vi "NEVSTOP QD Shortcuts.vi"(6 "Variant in":variant, 7 "Shift Pressed?":bool, 8 "error in (no error)":errorcluster, 10 "QD Combo Box Ref":refnum<vi>, 11 "QD Launch VI Ref":refnum<vi>) -> (0 "error out":errorcluster, 4 "Variant out":variant)   [LabVIEW 2017, in "NEVSTOP QD Shortcuts.lvlib"]
doc: "NEVSTOP Quickdrops. Using a choosing dialog for quick QD selection.\n\nDefault Shortcut - [Q]"
uses:
  NEVSTOP QD Shortcuts.lvlib
panel:
  in  "Undo Name":string="NESTOP Shortcuts"
  # "Do not change the connector pane of this VI.\n\nSee the block diagram for directions on how to use this template."
  # "Specify the name of the Undo transaction"
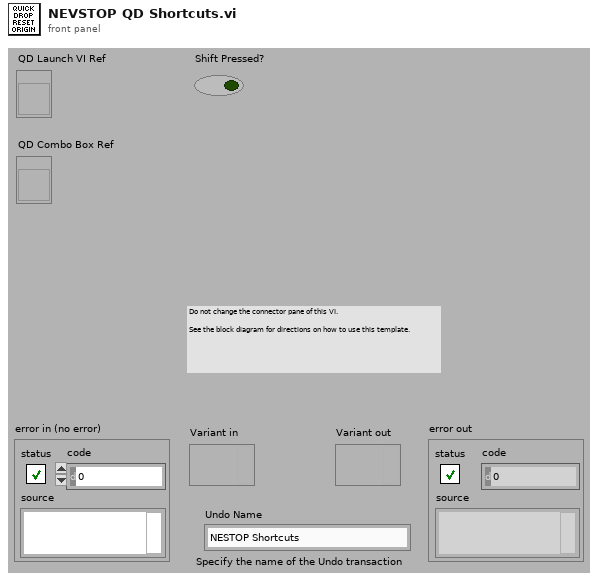
[diagram p1: front panel]
types:
  T1 = typedef "QuickDrop QDKS Info.ctl" = cluster{"VI Name":string, "VI Path":path, "Default Shortcut":string, "Assigned Shortcut":string, "Description":string}
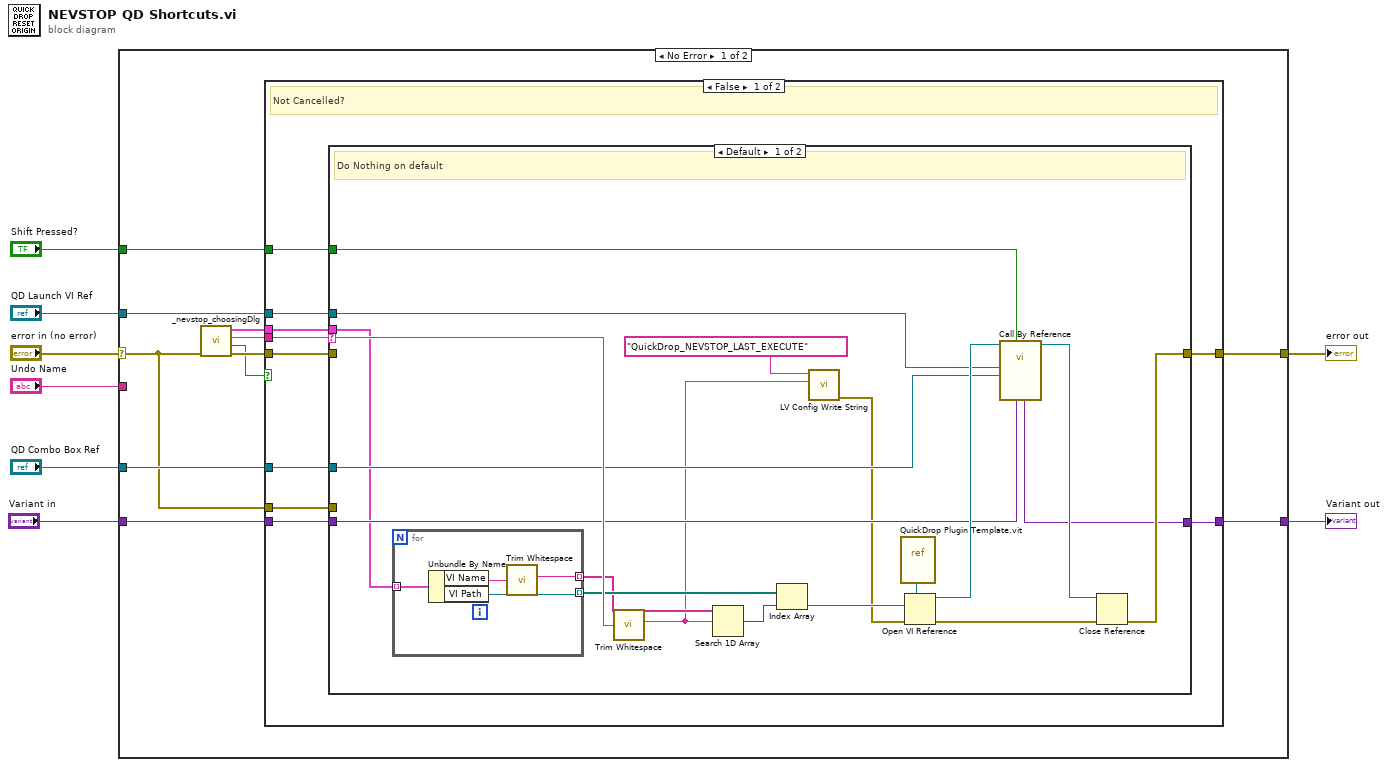
[diagram p0: block diagram]
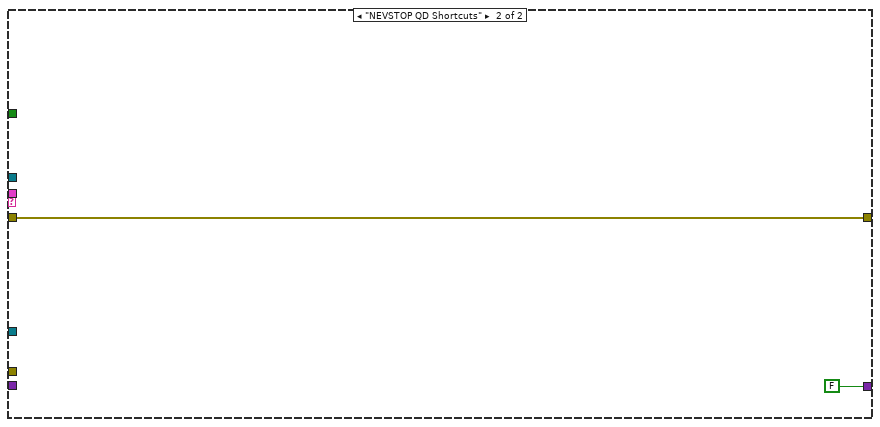
[diagram p2: hidden frame]
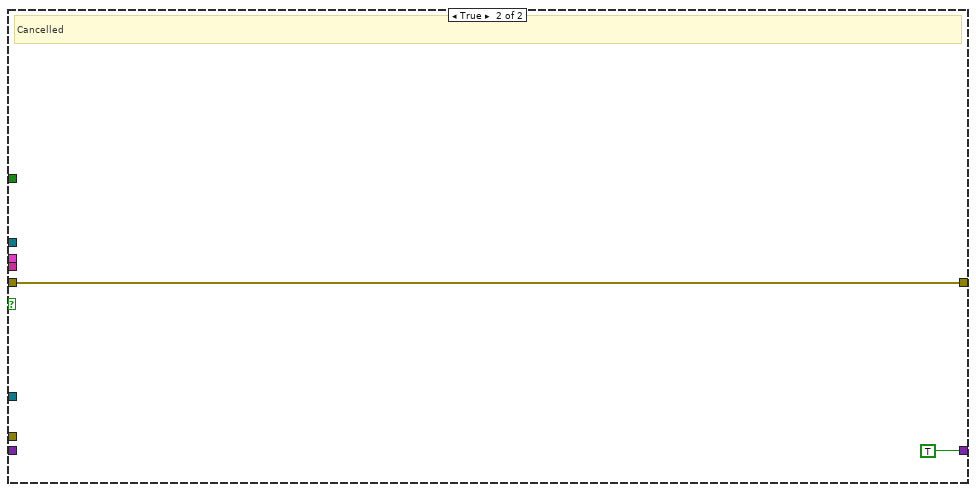
[diagram p3: hidden frame]
diagram:
  n1 = case shown="No Error" "error in (no error)" {
    selector: "error in (no error)" -> [w10 w57]
    tunnel: [w14 w57] -> w7
    tunnel: "QD Launch VI Ref" -> [w13 _]
    tunnel: "Shift Pressed?" -> [w17 _]
    tunnel: "QD Combo Box Ref" -> [w16 _]
    tunnel: "Variant in" -> [w12 _]
    tunnel: "Undo Name" -> [_ _]
    tunnel: [w11 _] -> w1
    frame No Error {
      n2 = call "_nevstop_choosingDlg.vi"("error in (no error)"=w10) -> ("error out"=w18:errorcluster, "Cancelled?"=w15:bool, "QuckDrop"=w19:string, "QDKS Info"=w9:T1[])  [unwired: 6 in, 1 out]
      n3 = case shown="False" w15 {
        tunnel: w19 -> [w29 _]
        tunnel: w18 -> [w28 w56]
        tunnel: w17 -> [w27 _]
        tunnel: w16 -> [w26 _]
        tunnel: [w25 w56] -> w14
        tunnel: w13 -> [w24 _]
        tunnel: w12 -> [w23 _]
        tunnel: [w22 TRUE] -> w11
        tunnel: w10 -> [w21 _]
        tunnel: w9 -> [w20 _]
        frame False {
          # "Not Cancelled?"
          n4 = case shown="Default" w29 {
            selector: w29 -> [w47 _]
            tunnel: w28 -> [_ w54]
            tunnel: w27 -> [w37 _]
            tunnel: w26 -> [w38 _]
            tunnel: [w41 w54] -> w25
            tunnel: w24 -> [w39 _]
            tunnel: w23 -> [w40 _]
            tunnel: [w36 FALSE] -> w22
            tunnel: w21 -> [_ _]
            tunnel: w20 -> [w33 _]
            frame Default {
              # "Do Nothing on default"
              n5 = for {
                tunnel: w33 -> [w52] mode=indexing
                tunnel: [w49] -> w34 mode=indexing
                tunnel: [w50] -> w46 mode=indexing
                n6 = Unbundle By Name(w52) -> ("VI Name"=w51:string, "VI Path"=w50:path)
                n7 = call-poly <vilib>:"Trim Whitespace.vi"("string"=w51) -> ("trimmed string"=w49:string)  [unwired: 1 in]
              }
              n8 = call-poly <vilib>:"Trim Whitespace.vi"("string"=w47) -> ("trimmed string"=w31:string)  [unwired: 1 in]
              n9 = Search 1D Array(1D array=w34, element=w31) -> (index of element=w45:i32)  [unwired: 1 in]
              n10 = Index Array(array=w46, index=w45) -> (element=w44:path)
              n11 = call <resource>:"LV Config Write String.vi"("value"=w31, "key"="QuickDrop_NEVSTOP_LAST_EXECUTE") -> ("error out"=w30:errorcluster)  [unwired: 5 in]
              n12 = vi-ref <resource>:"QuickDrop Plugin Template.vit"() -> (w48:refnum<vi>)
              n13 = Open VI Reference(type specifier VI Refnum (for type only)=w48, vi path=w44, error in (no error)=w30) -> (vi reference=w43:refnum<vi>, error out=w35:errorcluster)  [unwired: 3 in]
              n14 = call-by-ref "?"(reference=w43, "Variant in"=w40, "Shift Pressed?"=w37, "QD Combo Box Ref"=w38, "QD Launch VI Ref"=w39) -> (reference out=w42:refnum<vi>, "Variant out"=w36:variant)  [unwired: 7 in, 2 out]
              n15 = Close Reference(reference=w42, error in (no error)=w35) -> (error out=w41:errorcluster)
            }
            frame "NEVSTOP QD Shortcuts" {
            }
          }
        }
        frame True {
          # "Cancelled"
        }
      }
    }
    frame Error {
    }
  }
  "error out" <- w7
  "Variant out" <- w1
